vi "Discrete Moments.vi"   [LabVIEW 2020, in "NI_Gmath.lvlib"]
doc: "Returns the expected mean and variance of the random variate X, where X describes the selected distribution type. You must manually select the polymorphic instance to use."
uses:
  <vilib>/gmath/NI_Gmath.lvlib
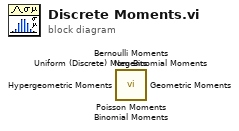
[diagram p0: block diagram]
diagram:
  n1 = call <vilib>:"Poisson Moments.vi"() -> ()  [unwired: 9 in, 3 out]
  n2 = call <vilib>:"Neg Binomial Moments.vi"() -> ()  [unwired: 9 in, 3 out]
  n3 = call <vilib>:"Hypergeometric Moments.vi"() -> ()  [unwired: 9 in, 3 out]
  n4 = call <vilib>:"Geometric Moments.vi"() -> ()  [unwired: 9 in, 3 out]
  n5 = call <vilib>:"Binomial Moments.vi"() -> ()  [unwired: 9 in, 3 out]
  n6 = call <vilib>:"Bernoulli Moments.vi"() -> ()  [unwired: 9 in, 3 out]
  n7 = call <vilib>:"Uniform (Discrete) Moments.vi"() -> ()  [unwired: 9 in, 3 out]
